vi "SV UFF58 ASCII Open File.vi"(0 "UFF58 file path":path, 5 "open mode (create:0)":enum16{"create ", "create or replace"}(ring), 11 "error in (no error)":errorcluster) -> (4 "refnum out":refnum<file>, 6 "UFF58 file path out":path, 15 "error out":errorcluster)   [LabVIEW 2017, in "SoundVib_UFF58.lvlib"]
doc: "Opens an existing UFF58 (universal file format) file, creates a new UFF58 file, or replaces an existing UFF file. You can input the file programmatically or interactively using a file dialog box."
uses:
  <vilib>/addons/Sound and Vibration/svt_UFF58/SoundVib_UFF58.lvlib
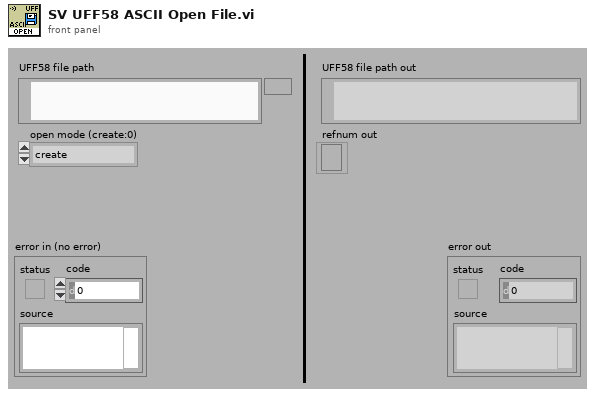
[diagram p1: front panel]
types:
  T1 = enum16{"existing file", "new file", "new or existing file", "existing dir", "new dir", "new or existing dir"}[]
  T2 = enum16{"open", "replace", "create", "open or create", "replace or create", "replace or create with confirmation"}
  T3 = enum16{"existing file", "new file", "new or existing file", "existing dir", "new dir", "new or existing dir"}
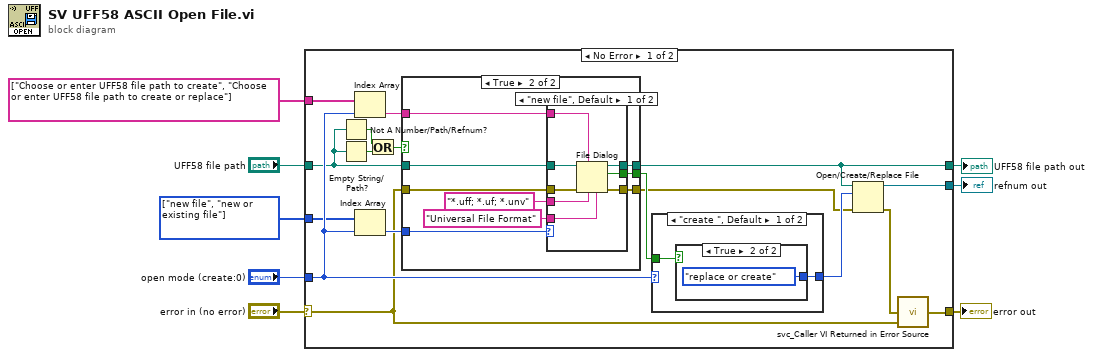
[diagram p0: block diagram]
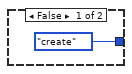
[diagram p2: hidden frame]
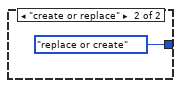
[diagram p3: hidden frame]
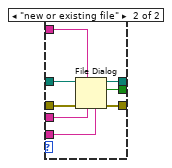
[diagram p5: hidden frame]
diagram:
  w1 = T1 [enum."new file", enum."new or existing file"] items=["existing file", "new file", "new or existing file", "existing dir", "new dir", "new or existing dir"]
  n1 = case shown="No Error" "error in (no error)" {
    selector: "error in (no error)" -> [w13 w59]
    tunnel: "UFF58 file path" -> [w18 w58]
    tunnel: "open mode (create:0)" -> [w22 _]
    tunnel: [w25 w59] -> w7
    tunnel: [w15 _] -> w6
    tunnel: [w16 w58] -> w3
    tunnel: string[] ["Choose or enter UFF58 file path to create", "Choose or enter UFF58 file path to create or replace"] -> [w10 _]
    tunnel: w1 -> [w9 _]
    frame No Error {
      n2 = Not A Number/Path/Refnum?(number/path/refnum=w18) -> (NaN/Path/Refnum?=w20:bool)
      n3 = Empty String/Path?(string/path=w18) -> (empty?=w19:bool)
      n4 = Index Array(array=w10, index=w22) -> (element=w21:string)
      n5 = Index Array(array=w9, index=w22) -> (element=w24:T3)
      n6 = Or(x=w20, y=w19) -> (x .or. y?=w17:bool)
      n7 = case shown="True" w17 {
        tunnel: w18 -> [w32 w37]
        tunnel: [w32 w41] -> w16
        tunnel: w24 -> [_ w35]
        tunnel: [_ w39] -> w23
        tunnel: w21 -> [_ w38]
        tunnel: w13 -> [w31 w34]
        tunnel: [w31 w33] -> w12
        frame False {
        }
        frame True {
          n8 = case shown="\"new file\", Default" w35 {
            tunnel: [w49 w57] -> w41
            tunnel: "Universal File Format" ("pattern label") -> [w48 w56]
            tunnel: [w44 w52] -> w39
            tunnel: w38 -> [w47 w55]
            tunnel: w37 -> [w46 w54]
            tunnel: "*.uff; *.uf; *.unv" ("pattern") -> [w45 w53]
            tunnel: w34 -> [w43 w51]
            tunnel: [w42 w50] -> w33
            frame "new file", Default {
              n9 = File Dialog(4:w48, 6:w45, 7:w47, 8:w43, 11:w46) -> (0:w42:errorcluster, 2:w44:bool, 3:w49:path)  [unwired: 2 in, 1 out]
            }
            frame "new or existing file" {
              n10 = File Dialog(4:w56, 6:w53, 7:w55, 8:w51, 11:w54) -> (0:w50:errorcluster, 2:w52:bool, 3:w57:path)  [unwired: 2 in, 1 out]
            }
          }
        }
      }
      n11 = case shown="\"create \", Default" w22 {
        tunnel: [w27 T2."replace or create" ("operation (0:open)")] -> w14
        tunnel: w23 -> [w26 _]
        frame "create ", Default {
          n12 = case shown="True" w26 {
            tunnel: [T2."create" ("operation (0:open)") T2."replace or create" ("operation (0:open)")] -> w27
            frame False {
            }
            frame True {
            }
          }
        }
        frame "create or replace" {
        }
      }
      n13 = Open/Create/Replace File(file path (use dialog)=w16, error in=w12, operation (0:open)=w14) -> (refnum out=w15:refnum<file>, error out=w11:errorcluster)  [unwired: 3 in, 1 out]
      n14 = call <vilib>:"svc_Caller VI Returned in Error Source.vi"("warning input to caller"=w13, "error in (no error)"=w11) -> ("error out"=w25:errorcluster)  [unwired: 3 in]
    }
    frame Error {
    }
  }
  "error out" <- w7
  "refnum out" <- w6
  "UFF58 file path out" <- w3
